vi "GetVelocity.vi"(8 "error in (no error)":errorcluster, 11 "VISA resource name":refnum<visa-resource-name>) -> (0 "error out":errorcluster, 2 "Velocity":dbl)   [LabVIEW 2012, in "Micos_uic.lvlib"]
doc: "Performs an instrument error query before terminating the software connection to the instrument."
uses:
  Micos_uic.lvlib
  <vilib>/Utility/error.llb/DialogType.ctl
  <vilib>/regexp/Match Regular Expression.xnode
panel:
  out "Read Buffer":string
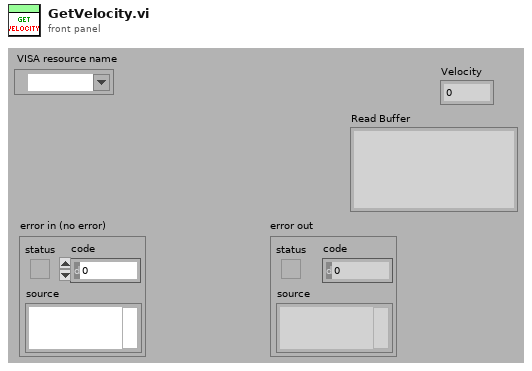
[diagram p1: front panel]
types:
  T1 = typedef "DialogType.ctl" = u16
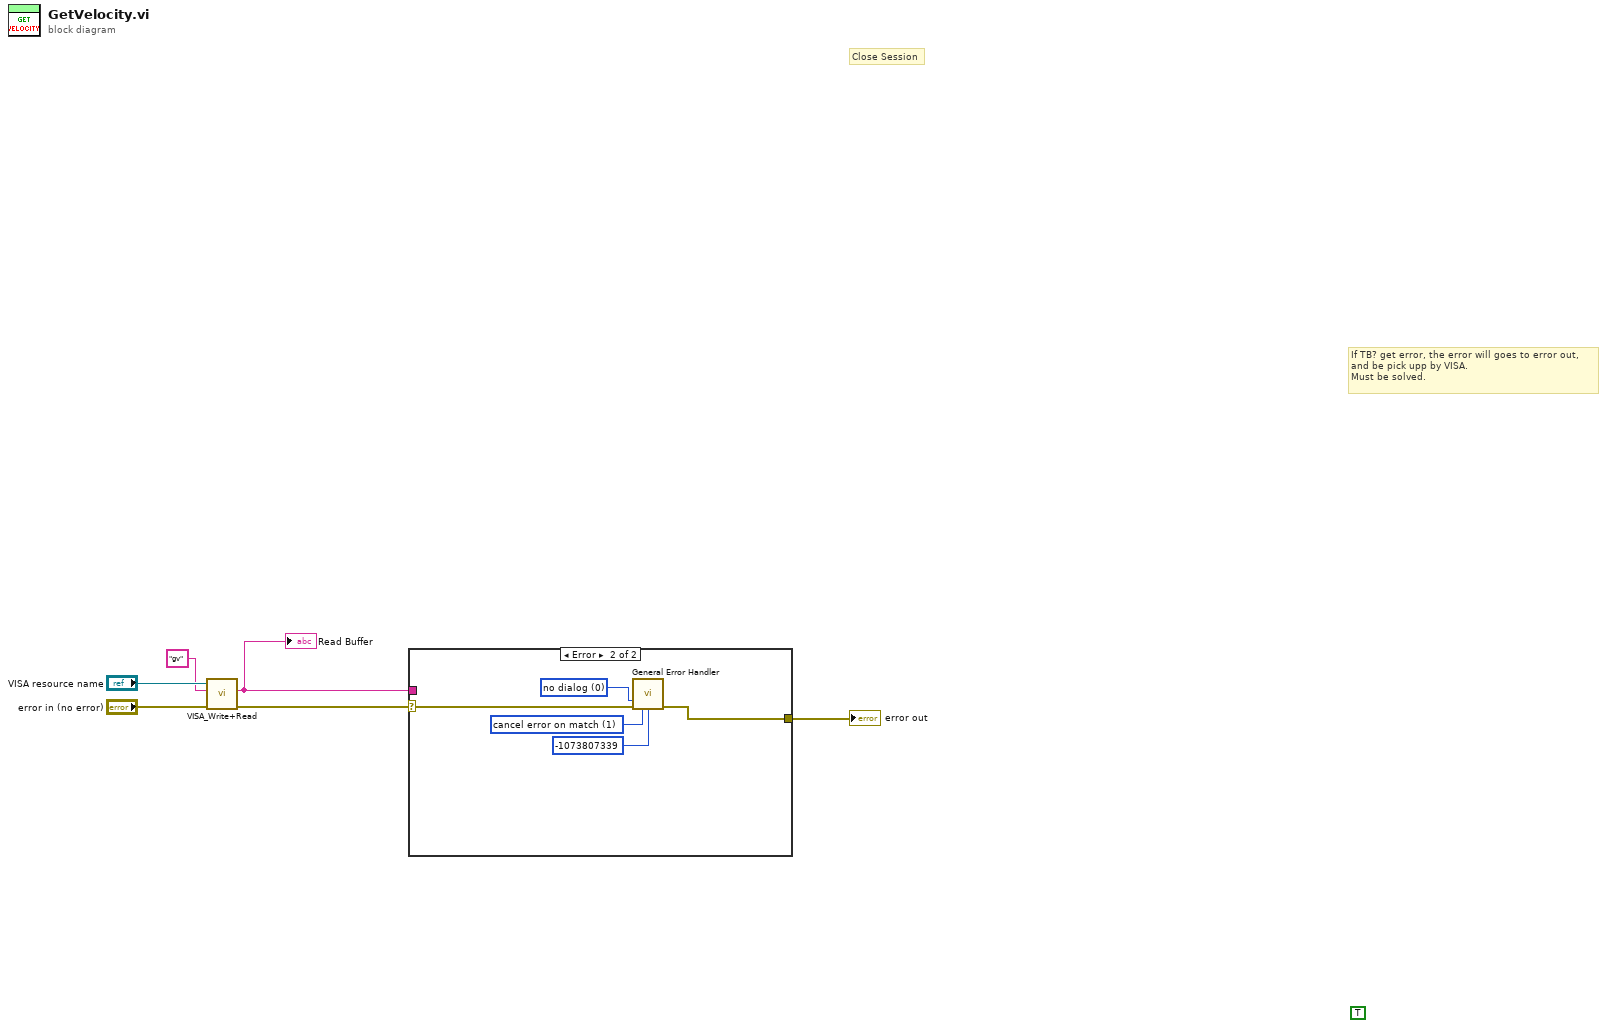
[diagram p0: block diagram]
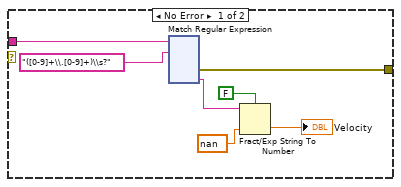
[diagram p2: hidden frame]
diagram:
  (unwired) TRUE
  # "If TB? get error, the error will goes to error out, \nand be pick upp by VISA.\nMust be solved."
  # "Close Session"
  n1 = call "VISA_Write+Read.vi"("error in (no error)"="error in (no error)", "Write Buffer"="gv" ("string"), "VISA resource name"="VISA resource name") -> ("error out"=w2:errorcluster, "readout"=w3:string)  [unwired: 6 in, 1 out]
  "Read Buffer" <- w3
  n2 = case shown="Error" w2 {
    selector: w2 -> [_ w129]
    tunnel: w3 -> [w10 _]
    tunnel: [w7 w128] -> w1
    frame No Error {
      n3 = xnode "Match Regular Expression"("input string"=w10, "regular expression"="([0-9]+\\.[0-9]+)\\s?") -> ("error out"=w7:errorcluster, "submatch 1"=w12:string)  [unwired: 4 in, 4 out]
      n4 = Fract/Exp String To Number(use system decimal point (T)=FALSE, string=w12, default (0 dbl)=nan ("default value 1")) -> (number=→"Velocity":dbl)  [unwired: 1 in, 1 out]
    }
    frame Error {
      w127 = T1 0 items=["no dialog", "OK message", "continue or stop message", "OK message + warnings", "continue/stop + warnings"] ("type of dialog (OK msg:1)")
      w131 = 1 items=["no exception", "cancel error on match", "set error on match"] ("[exception action] (none:0)")
      n5 = call <vilib>:"General Error Handler.vi"("type of dialog (OK msg:1)"=w127, "error in (no error)"=w129, "[exception action] (none:0)"=w131, "[exception code]"=-1073807339) -> ("error out"=w128:errorcluster)  [unwired: 7 in, 4 out]
    }
  }
  "error out" <- w1
